vi "Set target position.vi"(8 "error in (no error)":errorcluster, 10 "target position":dbl[](array[numeric]), 11 "StageSPIM in":refnum<class "StageSPIM.lvclass">) -> (0 "error out":errorcluster, 3 "StageSPIM out":refnum<class "StageSPIM.lvclass">)   [LabVIEW 2012, in "StageSPIM.lvclass"]
uses:
  StageSPIM.lvclass
  StageSPIM.lvclass/StageSPIM.ctl
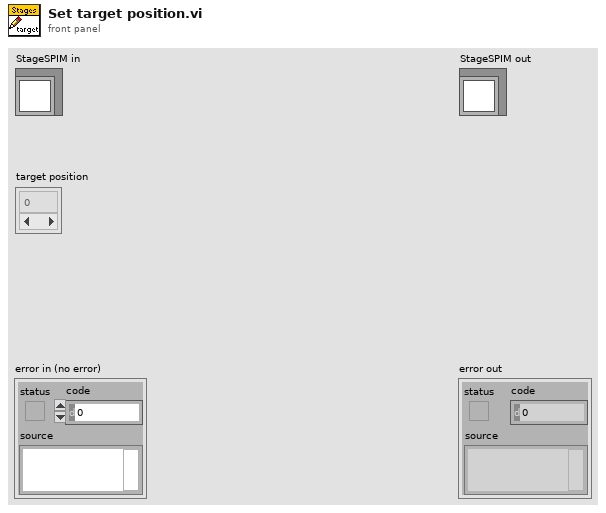
[diagram p1: front panel]
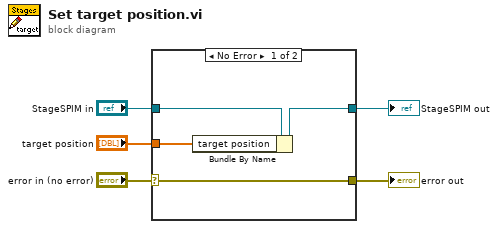
[diagram p0: block diagram]
diagram:
  n1 = case shown="No Error" "error in (no error)" {
    selector: "error in (no error)" -> [w9 w11]
    tunnel: [w9 w11] -> w4
    tunnel: [w7 w10] -> w2
    tunnel: "StageSPIM in" -> [w8 w10]
    tunnel: "target position" -> [w6 _]
    frame No Error {
      n2 = Bundle By Name(cluster=w8, "target position"=w6) -> (w7:refnum<class "StageSPIM.lvclass">)
    }
    frame Error {
    }
  }
  "error out" <- w4
  "StageSPIM out" <- w2
